vi "Write ic type.vi"(8 "error in (no error)":errorcluster caption="에러 입력(에러 없음)", 10 "ic type":T1, 11 "Haptic IC 입력":refnum<class "Haptic IC.lvclass">) -> (0 "error out":errorcluster caption="에러 출력", 3 "Haptic IC 출력":refnum<class "Haptic IC.lvclass">)   [LabVIEW 2020, in "Haptic IC.lvclass"]
uses:
  Haptic IC.lvclass
  Controls/(Ctrl)IC Type.ctl
  Haptic IC.lvclass/Haptic IC.ctl
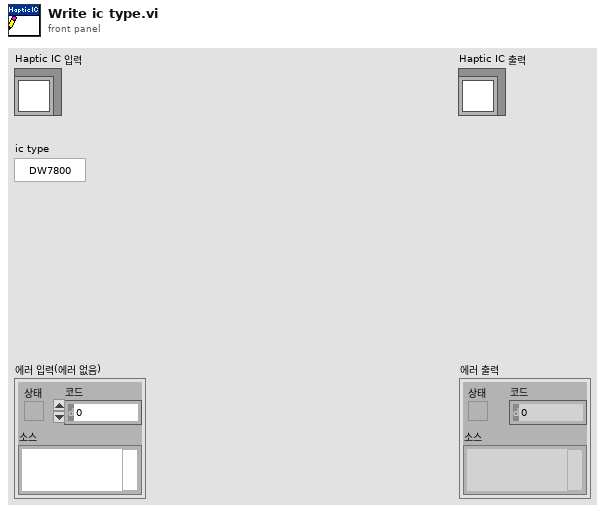
[diagram p1: front panel]
types:
  T1 = typedef "Haptic IC.lvclass/(Ctrl)IC Type.ctl" = enum8{"DW7800", "DW7802", "DW7912", "DW7914"}
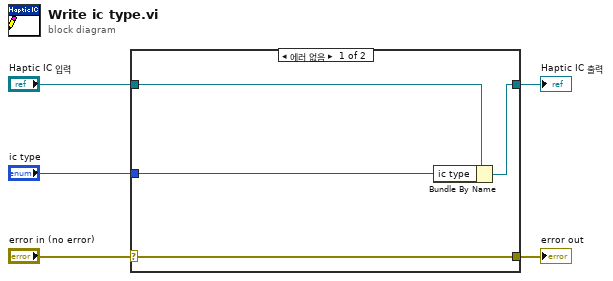
[diagram p0: block diagram]
diagram:
  n1 = case shown="에러 없음" "error in (no error)" {
    selector: "error in (no error)" -> [w9 w10]
    tunnel: [w9 w10] -> w4
    tunnel: [w7 w11] -> w2
    tunnel: "Haptic IC 입력" -> [w8 w11]
    tunnel: "ic type" -> [w6 _]
    frame No Error {
      n2 = Bundle By Name(cluster=w8, "ic type"=w6) -> (w7:refnum<class "Haptic IC.lvclass">)
    }
    frame Error {
    }
  }
  "error out" <- w4
  "Haptic IC 출력" <- w2
